vi "Pilot Control - Data.vi"(6 "Operation":enum16{"Init", "Get", "Set"}(ring)=enum."Get", 10 "Data in":i32) -> (2 "Data out":i32)   [LabVIEW 2021]
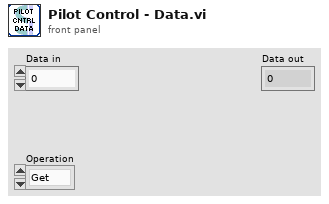
[diagram p1: front panel]
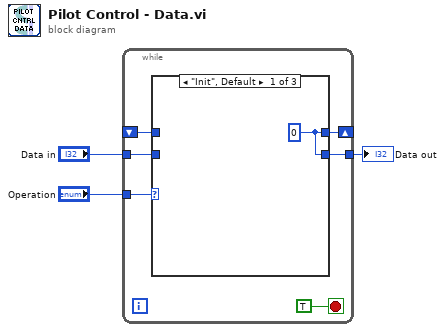
[diagram p0: block diagram]
diagram:
  n1 = while {
    tunnel: "Operation" -> [w8]
    shift-right: [w7] -> _
    shift-left: _ -> [w6]
    tunnel: [w5] -> w2
    tunnel: "Data in" -> [w4]
    stop <- TRUE stop-if-true
    n2 = case shown="\"Init\", Default" w8 {
      tunnel: [w10 w11 w12] -> w7
      tunnel: w6 -> [_ w11 _]
      tunnel: [w10 w11 w12] -> w5
      tunnel: w4 -> [_ _ w12]
      frame "Init", Default {
        w10 = 0
      }
      frame "Get" {
      }
      frame "Set" {
      }
    }
  }
  "Data out" <- w2
